vi "GUI_ECS_Dump_Reader.vi"() -> ()   [LabVIEW 2013]
uses:
  <vilib>/Utility/config.llb/Read Key (String).vi
  <vilib>/Utility/config.llb/NI_LVConfig.lvlib
panel:
  out "OAP Motor Positions":string[](array[string])
  out "Names":string[](array[string])
  in  "Multicolumn Listbox":i32(listbox)
  out "error out":errorcluster
  out "Array":string[][](array[string])
  in  "error in (no error)":errorcluster
  in  "configuration file path":path
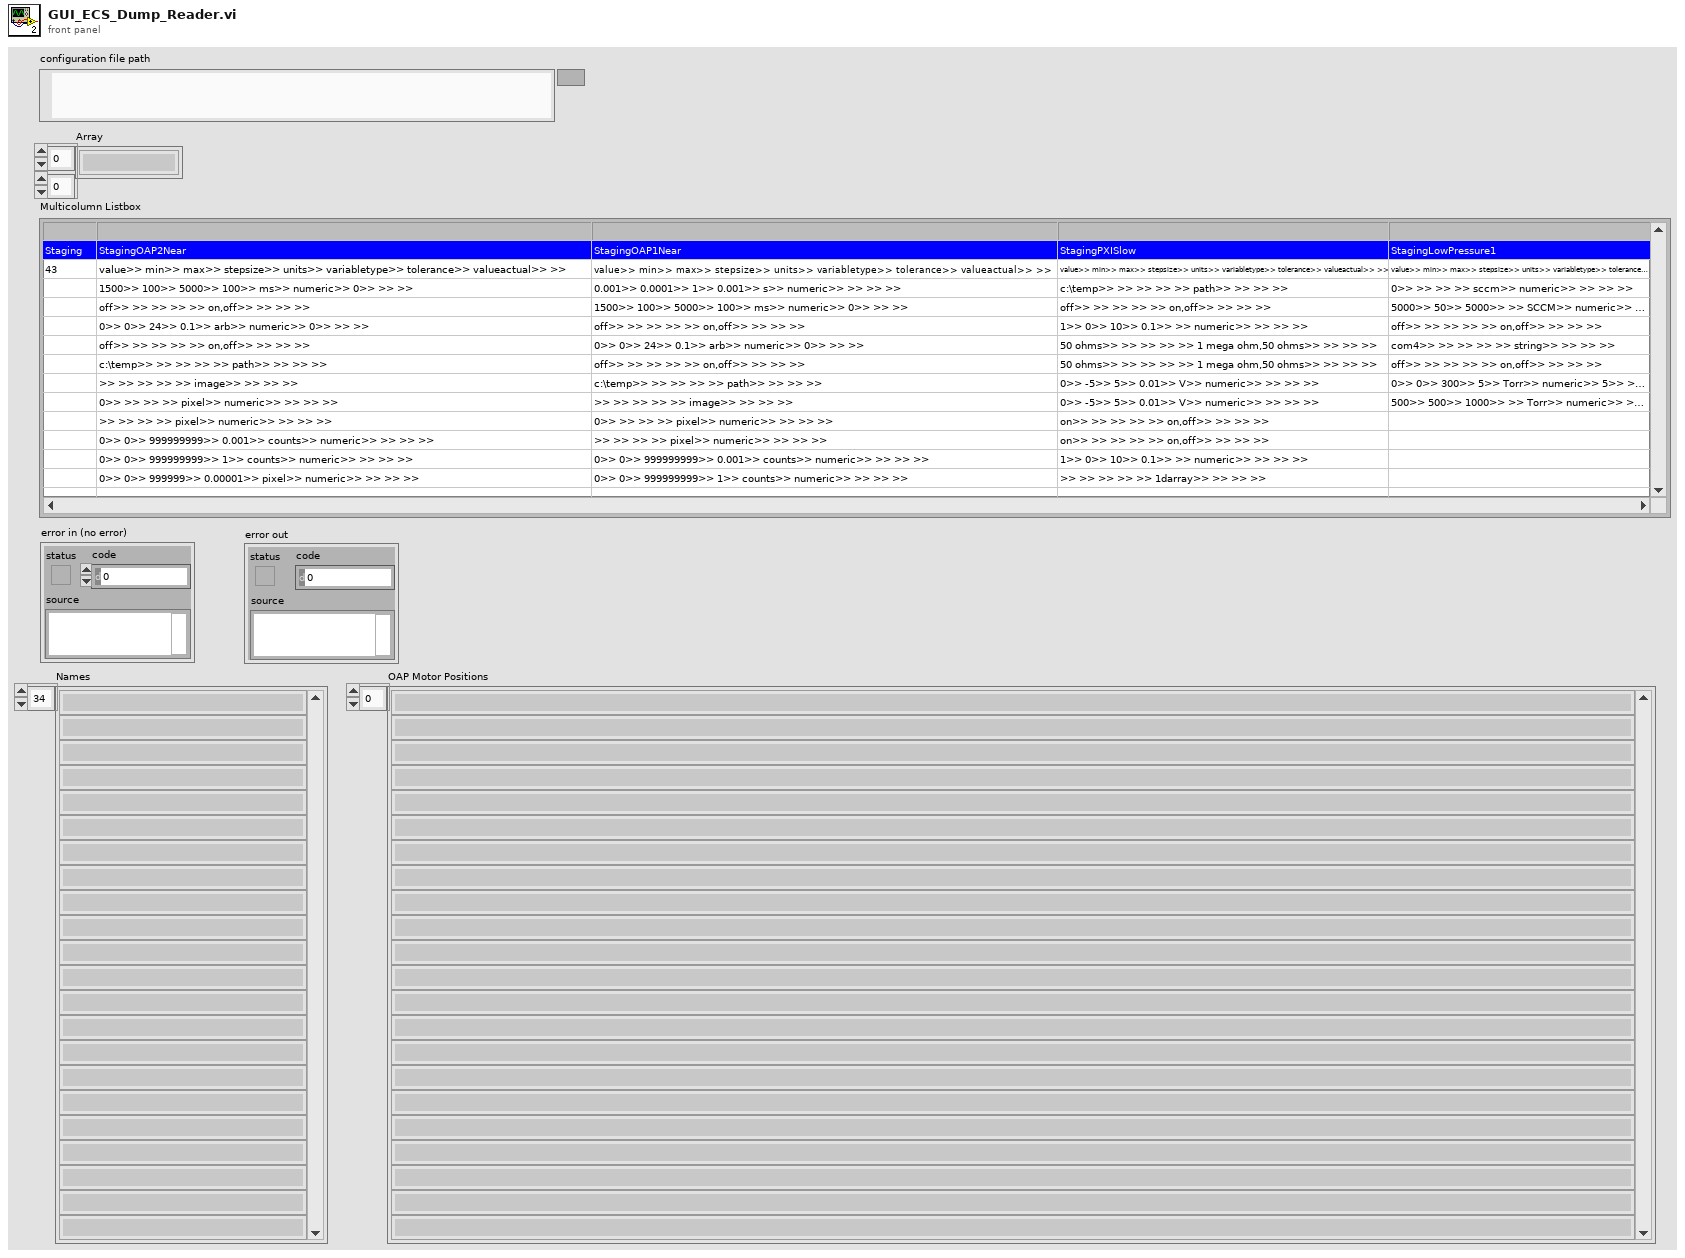
[diagram p1: front panel]
types:
  T1 = typedef "NI_LVConfig.lvlib/Config Data RefNum.ctl" = refnum<k1>
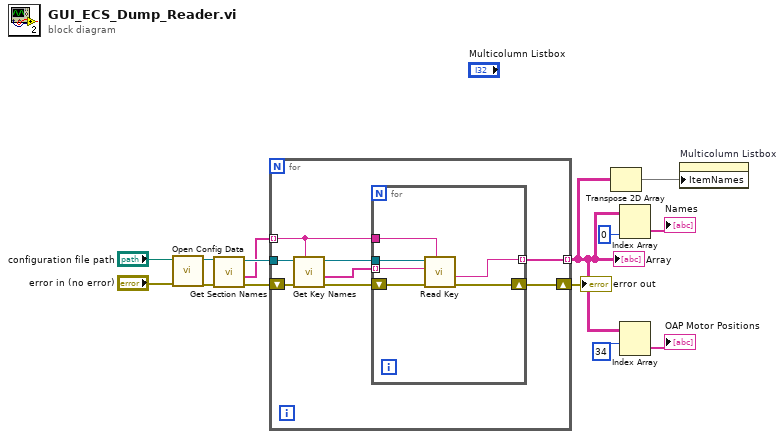
[diagram p0: block diagram]
diagram:
  n1 = call <vilib>:"Open Config Data.vi"("error in (no error)"="error in (no error)", "configuration file path"="configuration file path") -> ("error out"=w10:errorcluster, "refnum"=w13:T1)  [unwired: 7 in, 1 out]
  n2 = call <vilib>:"Get Section Names.vi"("error in (no error)"=w10, "refnum"=w13) -> ("error out"=w9:errorcluster, "section names"=w11:string[], "refnum out"=w12:T1)  [unwired: 7 in]
  n3 = for {
    tunnel: w12 -> [w22]
    tunnel: w11 -> [w18] mode=indexing
    shift-right: [w16] -> w7
    shift-left: w9 -> [w21]
    tunnel: [w15] -> w2 mode=indexing
    n4 = call <vilib>:"Get Key Names.vi"("section"=w18, "error in (no error)"=w21, "refnum"=w22) -> ("error out"=w17:errorcluster, "key names"=w19:string[], "refnum out"=w20:T1)  [unwired: 5 in, 1 out]
    n5 = for {
      tunnel: w20 -> [w28]
      tunnel: w19 -> [w27] mode=indexing
      tunnel: w18 -> [w26]
      tunnel: [w25] -> w15 mode=indexing
      shift-right: [w23] -> w16
      shift-left: w17 -> [w24]
      n6 = call-poly <vilib>:"Read Key.vi"("section"=w26, "error in (no error)"=w24, "key"=w27, "refnum"=w28) -> ("error out"=w23:errorcluster, "value"=w25:string)  [unwired: 4 in, 2 out]
    }
  }
  "Array" <- w2
  "error out" <- w7
  n7 = Transpose 2D Array(2D array=w2) -> (transposed array=w6:string[][])
  n8 = Index Array(array=w2, index (col)=0 ("disabled index (col)")) -> (element=→"Names":string[])  [unwired: 1 in]
  n9 = Index Array(array=w2, index (row)=34 ("disabled index (col)")) -> (element=→"OAP Motor Positions":string[])  [unwired: 1 in]
  n10 = property on="Multicolumn Listbox" class="MCListbox (strict)"("ItemNames"=w6) -> ()  [unwired: 2 in, 2 out]
